vi "Keithley 2400 Test.vi"() -> ()   [LabVIEW 2019]
panel:
  out "number":dbl
  in  "Send Read Command":bool
  out "return count":u32
  out "read buffer":string
  in  "Read Command String":string
  in  "Send Command":bool
  in  "Command String":string
  in  "Stop Read Loop":bool
  in  "Stop Command Loop":bool
  in  "On/Off":bool=TRUE
  in  "Change State":bool
  in  "Stop On/Off Loop":bool
  in  "Stop Init. Loop":bool
  in  "Initialize":bool
  out "error out":errorcluster
  in  "VISA Refnum in":refnum<visa-resource-name>
  in  "error in (no error)":errorcluster
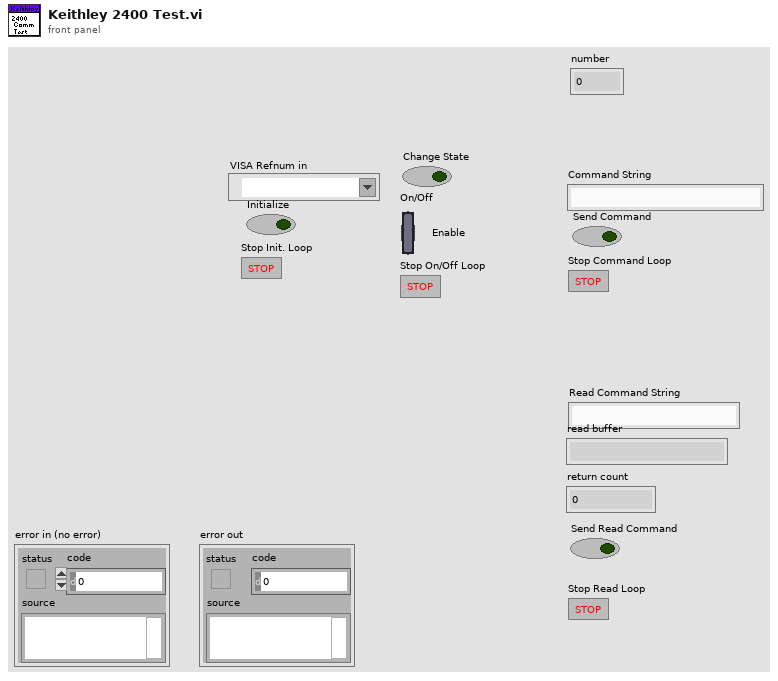
[diagram p1: front panel]
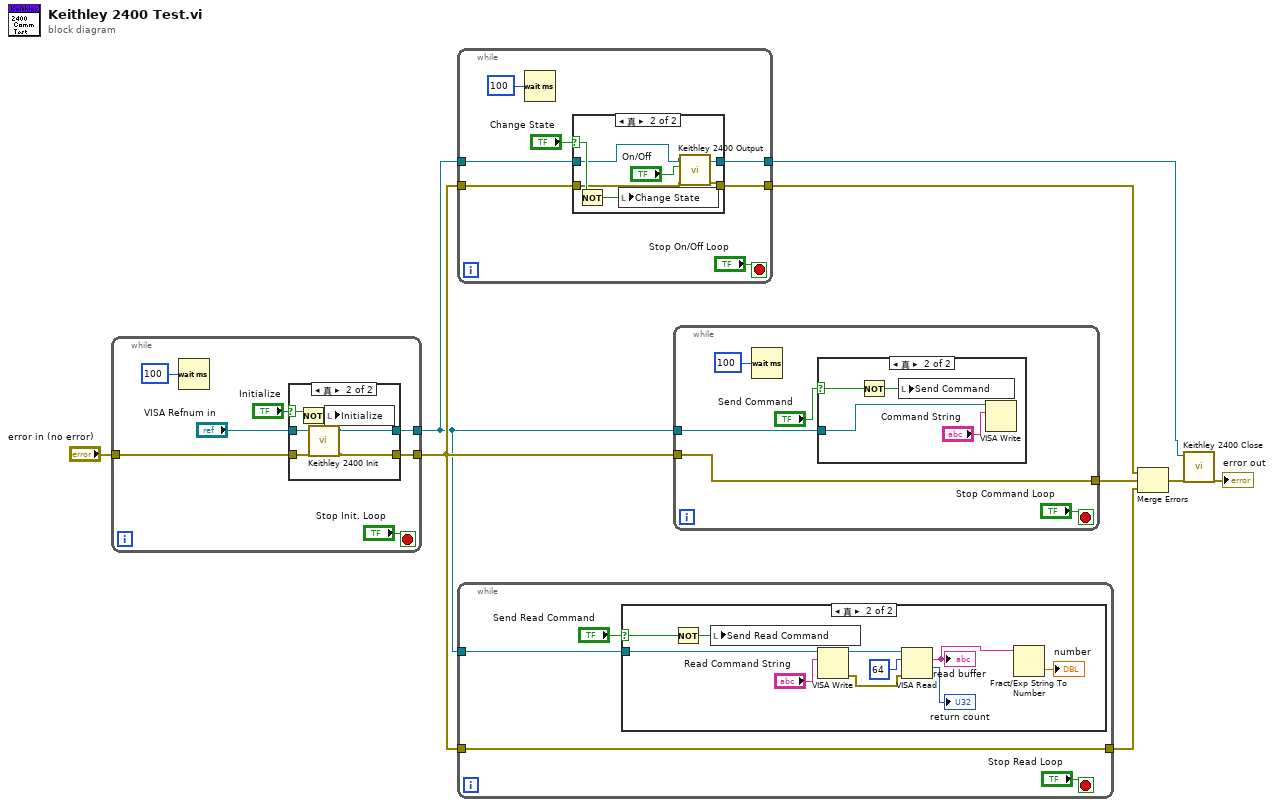
[diagram p0: block diagram]
diagram:
  n1 = while {
    tunnel: "error in (no error)" -> [w16]
    tunnel: [w11] -> w4
    tunnel: [w10] -> w8
    stop <- "Stop Init. Loop" stop-if-true
    n2 = Wait (ms)(milliseconds to wait=u32 100) -> ()  [unwired: 1 out]
    n3 = case shown="真" "Initialize" {
      selector: "Initialize" -> [_ w24]
      tunnel: w16 -> [w17 w21]
      tunnel: "VISA Refnum in" -> [w18 w22]
      tunnel: [w18 w19] -> w11
      tunnel: [w17 w20] -> w10
      frame False {
      }
      frame True {
        n4 = Not(x=w24) -> (.not. x?=w23:bool)
        n5 = call "Keithley 2400 Init.vi"("error in (no error)"=w21, "VISA Refnum in"=w22) -> ("error out"=w20:errorcluster, "VISA Refnum out"=w19:refnum<visa-resource-name>)  [unwired: 8 in]
        n6 = local write "Initialize"(w23) -> ()
      }
    }
  }
  n7 = while {
    tunnel: [w31] -> w3
    tunnel: w4 -> [w30]
    tunnel: w8 -> [w26]
    tunnel: [w25] -> w7
    stop <- "Stop On/Off Loop" stop-if-true
    n8 = Wait (ms)(milliseconds to wait=u32 100) -> ()  [unwired: 1 out]
    n9 = case shown="真" "Change State" {
      selector: "Change State" -> [_ w40]
      tunnel: [w33 w38] -> w31
      tunnel: w30 -> [w33 w35]
      tunnel: w26 -> [w32 w36]
      tunnel: [w32 w37] -> w25
      frame False {
      }
      frame True {
        n10 = Not(x=w40) -> (.not. x?=w39:bool)
        n11 = local write "Change State"(w39) -> ()
        n12 = call "Keithley 2400 Output.vi"("error in (no error)"=w36, "Enable Output (T: Enable)"="On/Off", "VISA resource name"=w35) -> ("error out"=w37:errorcluster, "VISA resource name out"=w38:refnum<visa-resource-name>)  [unwired: 7 in]
      }
    }
  }
  n13 = while {
    tunnel: w8 -> [w43]
    tunnel: [w43] -> w5
    tunnel: w4 -> [w42]
    stop <- "Stop Read Loop" stop-if-true
    n14 = case shown="真" "Send Read Command" {
      selector: "Send Read Command" -> [_ w53]
      tunnel: w42 -> [_ w52]
      frame False {
      }
      frame True {
        n15 = Not(x=w53) -> (.not. x?=w47:bool)
        n16 = local write "Send Read Command"(w47) -> ()
        n17 = VISA Write(VISA resource name=w52, write buffer="Read Command String") -> (VISA resource name out=w50:refnum<visa-resource-name>, error out=w49:errorcluster)  [unwired: 1 in, 1 out]
        n18 = VISA Read(VISA resource name=w50, byte count=u32 64, error in (no error)=w49) -> (read buffer=w46:string, return count=→"return count":u32)  [unwired: 2 out]
        "read buffer" <- w46
        n19 = Fract/Exp String To Number(string=w46) -> (number=→"number":dbl)  [unwired: 3 in, 1 out]
      }
    }
  }
  n20 = while {
    tunnel: w8 -> [w58]
    tunnel: [w58] -> w6
    tunnel: w4 -> [w55]
    stop <- "Stop Command Loop" stop-if-true
    n21 = Wait (ms)(milliseconds to wait=u32 100) -> ()  [unwired: 1 out]
    n22 = case shown="真" "Send Command" {
      selector: "Send Command" -> [_ w62]
      tunnel: w55 -> [_ w60]
      frame False {
      }
      frame True {
        n23 = Not(x=w62) -> (.not. x?=w61:bool)
        n24 = local write "Send Command"(w61) -> ()
        n25 = VISA Write(VISA resource name=w60, write buffer="Command String") -> ()  [unwired: 1 in, 3 out]
      }
    }
  }
  n26 = Merge Errors(w7, w6, w5) -> (w2:errorcluster)
  n27 = call "Keithley 2400 Close.vi"("error in (no error)"=w2, "VISA Refnum in"=w3) -> ("error out"=→"error out":errorcluster)  [unwired: 9 in]
